vi "Rinocloud_HTTP_update_metadata.vi"(4 "parent ID":string, 5 "self ID":string, 6 "Extra metadata array":T1(array[cluster])=[{"Attribute"="", "Value"="", "Data type"=enum."<null>"}], 7 "Notes":string, 8 "Tags":string, 9 "Name":string) -> (0 "body":string, 1 "headers":string, 2 "ID":i32, 3 "Saved":bool)   [LabVIEW 2013]
uses:
  Rinocloud_global_variable.vi
  <vilib>/httpClient/POSTBuffer.vi
  <vilib>/httpClient/LabVIEWHTTPClient.lvlib
panel:
  out "error out":errorcluster
  out "JSON payload":string
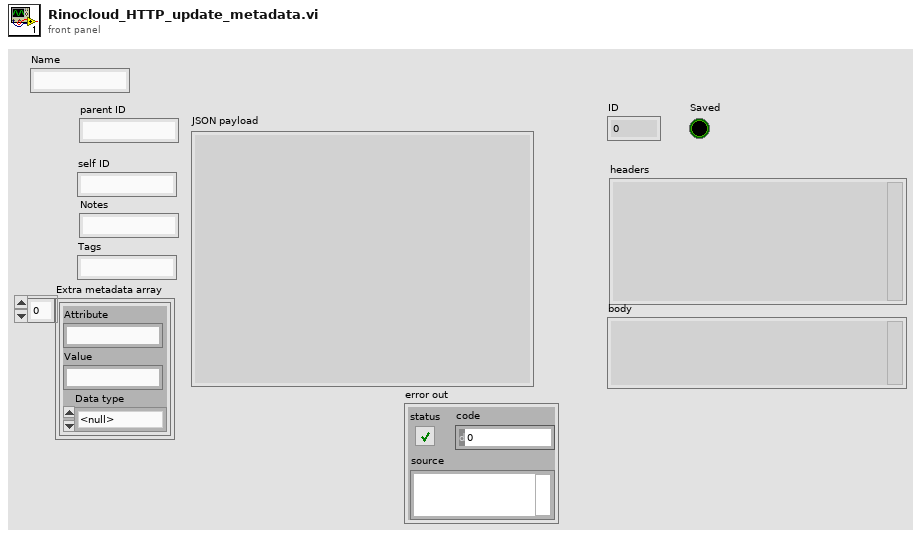
[diagram p1: front panel]
types:
  T1 = cluster{"Attribute":string, "Value":string, "Data type":enum16{"Numeric", "String", "1D array of strings", "1D array of doubles", "Data JSON string", "<null>"}}[]
  T2 = cluster{"Name":string, "Notes":string, "Tags":string}
  T3 = typedef "LabVIEWHTTPClient.lvlib/ClientHandle.ctl" = refnum<k1>
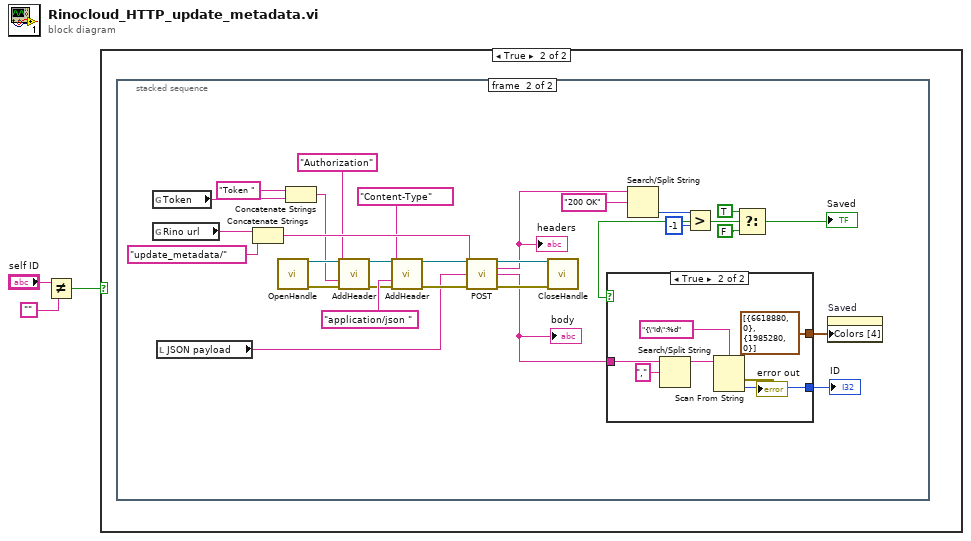
[diagram p0: block diagram]
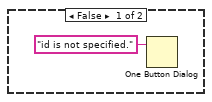
[diagram p2: hidden frame]
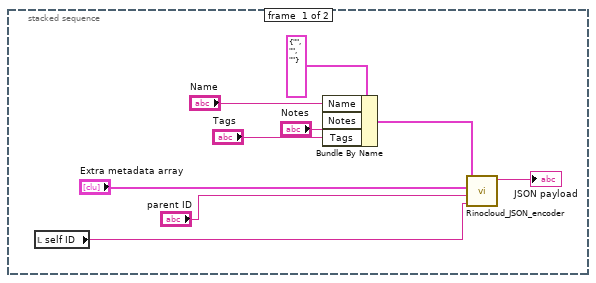
[diagram p3: hidden frame]
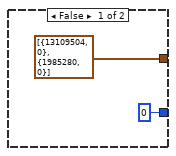
[diagram p4: hidden frame]
diagram:
  n1 = Not Equal?(x="self ID", y="") -> (x != y?=w1:bool)
  n2 = case shown="True" w1 {
    frame False {
      n3 = One Button Dialog(message="id is not specified.") -> ()  [unwired: 1 in, 1 out]
    }
    frame True {
      n4 = stacked-sequence {
        frame #0 {
          n5 = local read "self ID"() -> (w6:string)
          n6 = Bundle By Name(cluster=T2 {"Name"="", "Notes"="", "Tags"=""} ("Metadata"), "Name"="Name", "Notes"="Notes", "Tags"="Tags") -> (w10:T2)
          n7 = call "Rinocloud_JSON_encoder.vi"("self ID"=w6, "parent ID"="parent ID", "Extra metadata array"="Extra metadata array", "Metadata"=w10) -> ("JSON payload"=→"JSON payload":string)  [unwired: 7 in]
        }
        frame #1 {
          n8 = global read "Rinocloud_global_variable.vi" "Token"() -> (w34:string)
          n9 = global read "Rinocloud_global_variable.vi" "Rino url"() -> (w40:string)
          n10 = local read "JSON payload"() -> (w14:string)
          n11 = Concatenate Strings(w40, "update_metadata/" ("Combo Box 2")) -> (w42:string)
          n12 = call <vilib>:"OpenHandle.vi"() -> ("client handle out"=w38:T3, "error out"=w35:errorcluster)  [unwired: 14 in]
          n13 = Concatenate Strings("Token " ("value"), w34) -> (w36:string)
          n14 = call <vilib>:"AddHeader.vi"("client handle"=w38, "header"="Authorization" ("url"), "value"=w36, "error in (no error)"=w35) -> ("client handle out"=w18:T3, "error out"=w16:errorcluster)  [unwired: 10 in]
          n15 = call <vilib>:"AddHeader.vi"("client handle"=w18, "header"="Content-Type", "value"="application/json ", "error in (no error)"=w16) -> ("client handle out"=w17:T3, "error out"=w15:errorcluster)  [unwired: 10 in]
          n16 = call-poly <vilib>:"POST.vi"("client handle"=w17, "url"=w42, "buffer"=w14, "error in (no error)"=w15) -> ("client handle out"=w33:T3, "headers"=w21:string, "body"=w22:string, "error out"=w32:errorcluster)  [unwired: 8 in]
          "headers" <- w21
          "body" <- w22
          n17 = call <vilib>:"CloseHandle.vi"("client handle"=w33, "error in (no error)"=w32) -> ()  [unwired: 13 in, 1 out]
          n18 = Search/Split String(string=w21, search string/char (-)="200 OK") -> (offset of match=w30:i32)  [unwired: 1 in, 2 out]
          n19 = Greater?(x=w30, y=-1) -> (0:w28:bool)
          n20 = Select(t=TRUE, s=w28, f=FALSE) -> (s? t:f=w25:bool)
          "Saved" <- w25
          n21 = case shown="True" w25 {
            tunnel: w22 -> [_ w51]
            tunnel: [0 w47] -> w24
            tunnel: [cluster{u32, u32}[] [{13109504, 0}, {1985280, 0}] ("Colors [4]") cluster{u32, u32}[] [{6618880, 0}, {1985280, 0}] ("Colors [4]")] -> w23
            frame False {
            }
            frame True {
              n22 = Search/Split String(string=w51, search string/char (-)=",") -> (substring before match=w49:string)  [unwired: 1 in, 2 out]
              n23 = Scan From String(format string="{\"id\":%d", input string=w49) -> (error out=→"error out":errorcluster, output 1=w47:i32)  [unwired: 3 in, 2 out]
            }
          }
          "ID" <- w24
          n24 = property on="Saved" class="Bool (strict)"("Colors [4]"=w23) -> ()  [unwired: 2 in, 2 out]
        }
      }
    }
  }
